vi "TankDriveHandler.vi"(0 "TankDrive Queue":refnum<queue>, 5 "Left Motor Value":dbl, 7 "Right Motor Value":dbl, 9 "HalfSpeed (F)":bool, 11 "Error In (no error)":errorcluster, 12 "Sensitivity (.01)":dbl=0.01) -> (15 "Error Out":errorcluster)   [LabVIEW 2013]
doc: "Handles input for tank drive. \nParameters:\n- Motor values: default to 0 if unwired.\n- Mode: Init or Do. Init will set the motors to 0 and prepare this VI for future calls, so this VI should be called with Init first. Do will update the motor values according to LeftMotorValue and RightMotorValue.\n- HalfSpeed: If true, cuts motor speed in half. Defaults to false.\n- Sensitivity: A measure of how big a change in joystick value is needed to trigger an event. Defaults to .01.\n-TankDrive Queue: the queue on which instructions will be enqueued\nIf the motor values changed significantly, a tank drive enstruction will be enqueued."
uses:
  QueueInstruction.ctl
  SubsystemEnum.ctl
  ActionEnum.ctl
  TankDriveInstruction.ctl
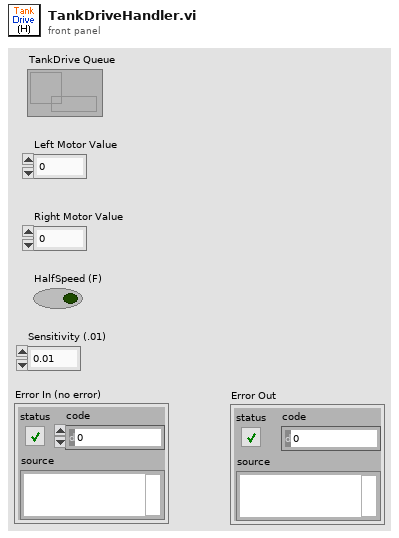
[diagram p1: front panel]
types:
  T1 = typedef "SubsystemEnum.ctl" = enum16{"TankDrive", "FirePneumatic", "Climber", "ClimbWeight", "ShooterAngle"}
  T2 = typedef "TankDriveInstruction.ctl" = cluster{"LeftMotorValue":dbl, "RightMotorValue":dbl, "HalfSpeed":bool}
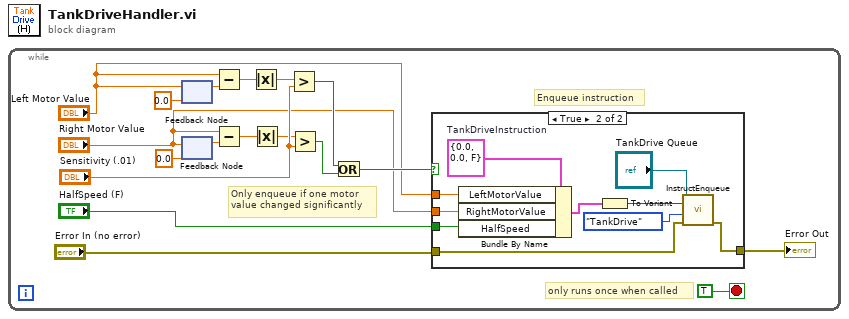
[diagram p0: block diagram]
diagram:
  n1 = while {
    stop <- TRUE stop-if-true
    # "Enqueue instruction"
    # "Only enqueue if one motor\nvalue changed significantly"
    # "only runs once when called"
    n2 = feedback #1(0.0) -> (w3:dbl)
    n3 = feedback-in #1("Left Motor Value") -> ()
    n4 = feedback-in #2("Right Motor Value") -> ()
    n5 = feedback #2(0.0) -> (w4:dbl)
    n6 = Subtract(x="Left Motor Value", y=w3) -> (x-y=w14:dbl)
    n7 = Subtract(x="Right Motor Value", y=w4) -> (x-y=w13:dbl)
    n8 = Absolute Value(x=w14) -> (abs(x)=w12:dbl)
    n9 = Absolute Value(x=w13) -> (abs(x)=w11:dbl)
    n10 = Greater?(x=w12, y="Sensitivity (.01)") -> (0:w9:bool)
    n11 = Greater?(x=w11, y="Sensitivity (.01)") -> (0:w10:bool)
    n12 = Or(x=w9, y=w10) -> (x .or. y?=w8:bool)
    n13 = case shown="True" w8 {
      tunnel: "Error In (no error)" -> [w19 w22]
      tunnel: "Right Motor Value" -> [_ w29]
      tunnel: [w19 w21] -> w7
      tunnel: "HalfSpeed (F)" -> [_ w28]
      tunnel: "Left Motor Value" -> [_ w20]
      frame False {
      }
      frame True {
        w27 = T2 {"LeftMotorValue"=0.0, "RightMotorValue"=0.0, "HalfSpeed"=FALSE}  # TankDriveInstruction
        n14 = Bundle By Name(cluster=w27, "LeftMotorValue"=w20, "RightMotorValue"=w29, "HalfSpeed"=w28) -> (w26:T2)
        n15 = To Variant(anything=w26) -> (Variant=w24:variant)
        n16 = call "InstructEnqueue.vi"("error in (no error)"=w22, "Subsystem"=SubsystemEnum."TankDrive", "Variant"=w24, "Queue"="TankDrive Queue") -> ("error out"=w21:errorcluster)  [unwired: 7 in]
      }
    }
    "Error Out" <- w7
  }
